vi "2 MissionHeadingGoodness.vi"(2 "Heading":dbl, 3 "Waypoint Location":T1 {"North" format="%#_10f"; "East" format="%#_8f"}, 4 "Waypoint in":refnum<class "Waypoint.lvclass">) -> (6 "Target Goodness":dbl, 7 "No-Go Goodness":dbl, 9 "Direction Change Goodness":dbl)   [LabVIEW 2011]
doc: "This VI simply runs the necessary components of the goodness function and outputs their \"goodness value\" for a specific test heading."
uses:
  2 Typedefs/UTM Location.ctl
  2 Classes/Waypoint/Waypoint.lvclass
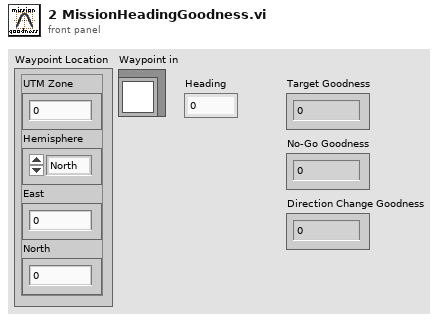
[diagram p1: front panel]
types:
  T1 = typedef "UTM Location.ctl" = cluster{"UTM Zone":dbl, "Hemisphere":enum16{"North", "South"}, "East":dbl, "North":dbl}
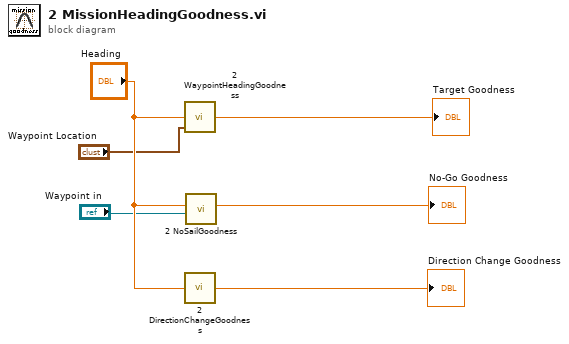
[diagram p0: block diagram]
diagram:
  n1 = call "2 WaypointHeadingGoodness.vi"("Waypoint Location"="Waypoint Location", "Heading to Test"="Heading") -> ("Goodness"=→"Target Goodness":dbl)  [unwired: 3 in]
  n2 = call "2 DirectionChangeGoodness.vi"("Test Heading"="Heading") -> ("Goodness"=→"Direction Change Goodness":dbl)
  n3 = call "2 NoSailGoodness.vi"("Waypoint in"="Waypoint in", "Heading to Test"="Heading") -> ("Goodness"=→"No-Go Goodness":dbl)  [unwired: 9 in]
